vi "Delta_RH.vi"() -> ()   [LabVIEW 2019]
uses:
  <vilib>/Analysis/baseanly.llb/Mean (DBL).vi
  DeltaRamp_globals.vi
  Global 2.vi
  B_Globals.vi
  <vilib>/Analysis/NI_AALBase.lvlib
panel:
  in  "RW Delay":i32=50
  out "Exec Time [ms]":u32
  in  "Reading Delay [ms]":i32=100 min=5
  out "read buffer":string
  in  "B/T":bool
  in  "Smart Avs":bool=TRUE
  in  "Points":dbl=1.0
  out "PpP":dbl
  in  "Combo Box":string(combo)
  in  "Save":bool
  in  "Abort Delta":bool
  out "B [T]":dbl=0.49837
  in  "Arm":bool
  in  "Measure":bool
  in  "Comp":dbl=10.0
  in  "Delay":dbl=0.002
  in  "I_Max":dbl=0.00055
  out "T":cluster{"X":dbl[], "Y":dbl[]}[](graph)=[{"X"=[0.48596000000030654, 0.48632999999976745, 0.4888800000004717, 0.4914299999991856, 0.49799999999988437, 0.49837000000048626, 0.49799999999964834, 0.49764000000059827, 0.4972699999998548, 0.49799999999964706, 0.4976400000005962, 0.4979999999996451, 0.49764000000114167, 0.4987299999995217, 0.49837000000048276, 0.4979999999996453, 0.49764000000060443, 0.4980000000000499, 0.4983700000004744, 0.4979999999996602, 0.4983700000001006, 0.4979999999996734, 0.49764000000018094, 0.4979999999996305, 0.4976400000006558, 0.4979999999996311, 0.4976399999998779, 0.49799999999967304, 0.4983699999999628, 0.49799999999964784, 0.49764000000002906, 0.4983699999999084, 0.49799999999967276, 0.498370000000109, 0.4979999999996426, 0.4983700000001016, 0.4979999999996246, 0.4983700000001098, 0.4979999999996428, 0.4976400000006453], "Y"=[nan, nan, nan, nan, nan, nan, nan, nan, nan, nan, nan, nan, nan, nan, nan, nan, nan, nan, nan, nan, nan, nan, nan, nan, nan, nan, nan, nan, nan, nan, nan, nan, nan, nan, nan, nan, nan, nan, nan, nan]}] caption="XY Graph"
  in  "Reset":bool
  out "Spl T [K]":dbl=6.1992
  out "R [Ohm]":dbl=nan
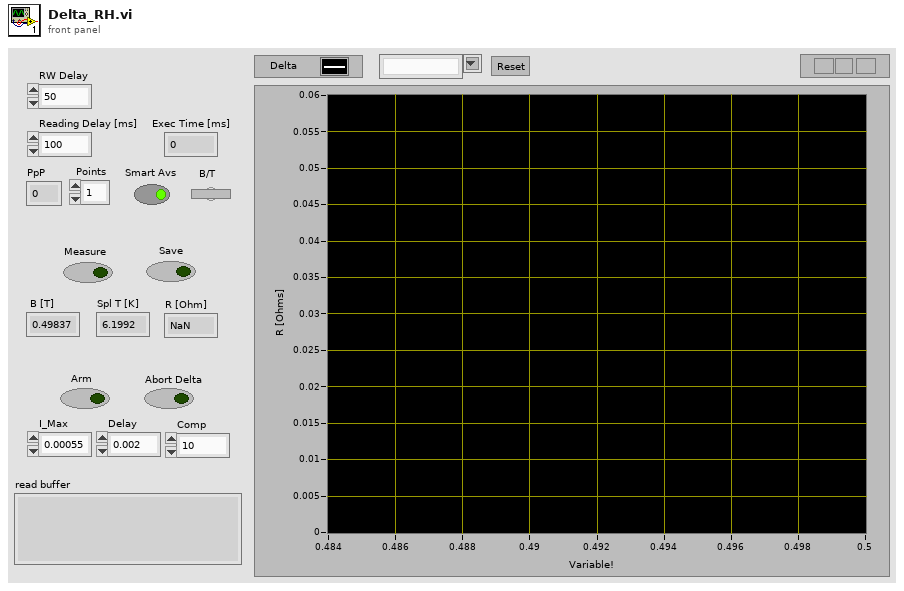
[diagram p1: front panel]
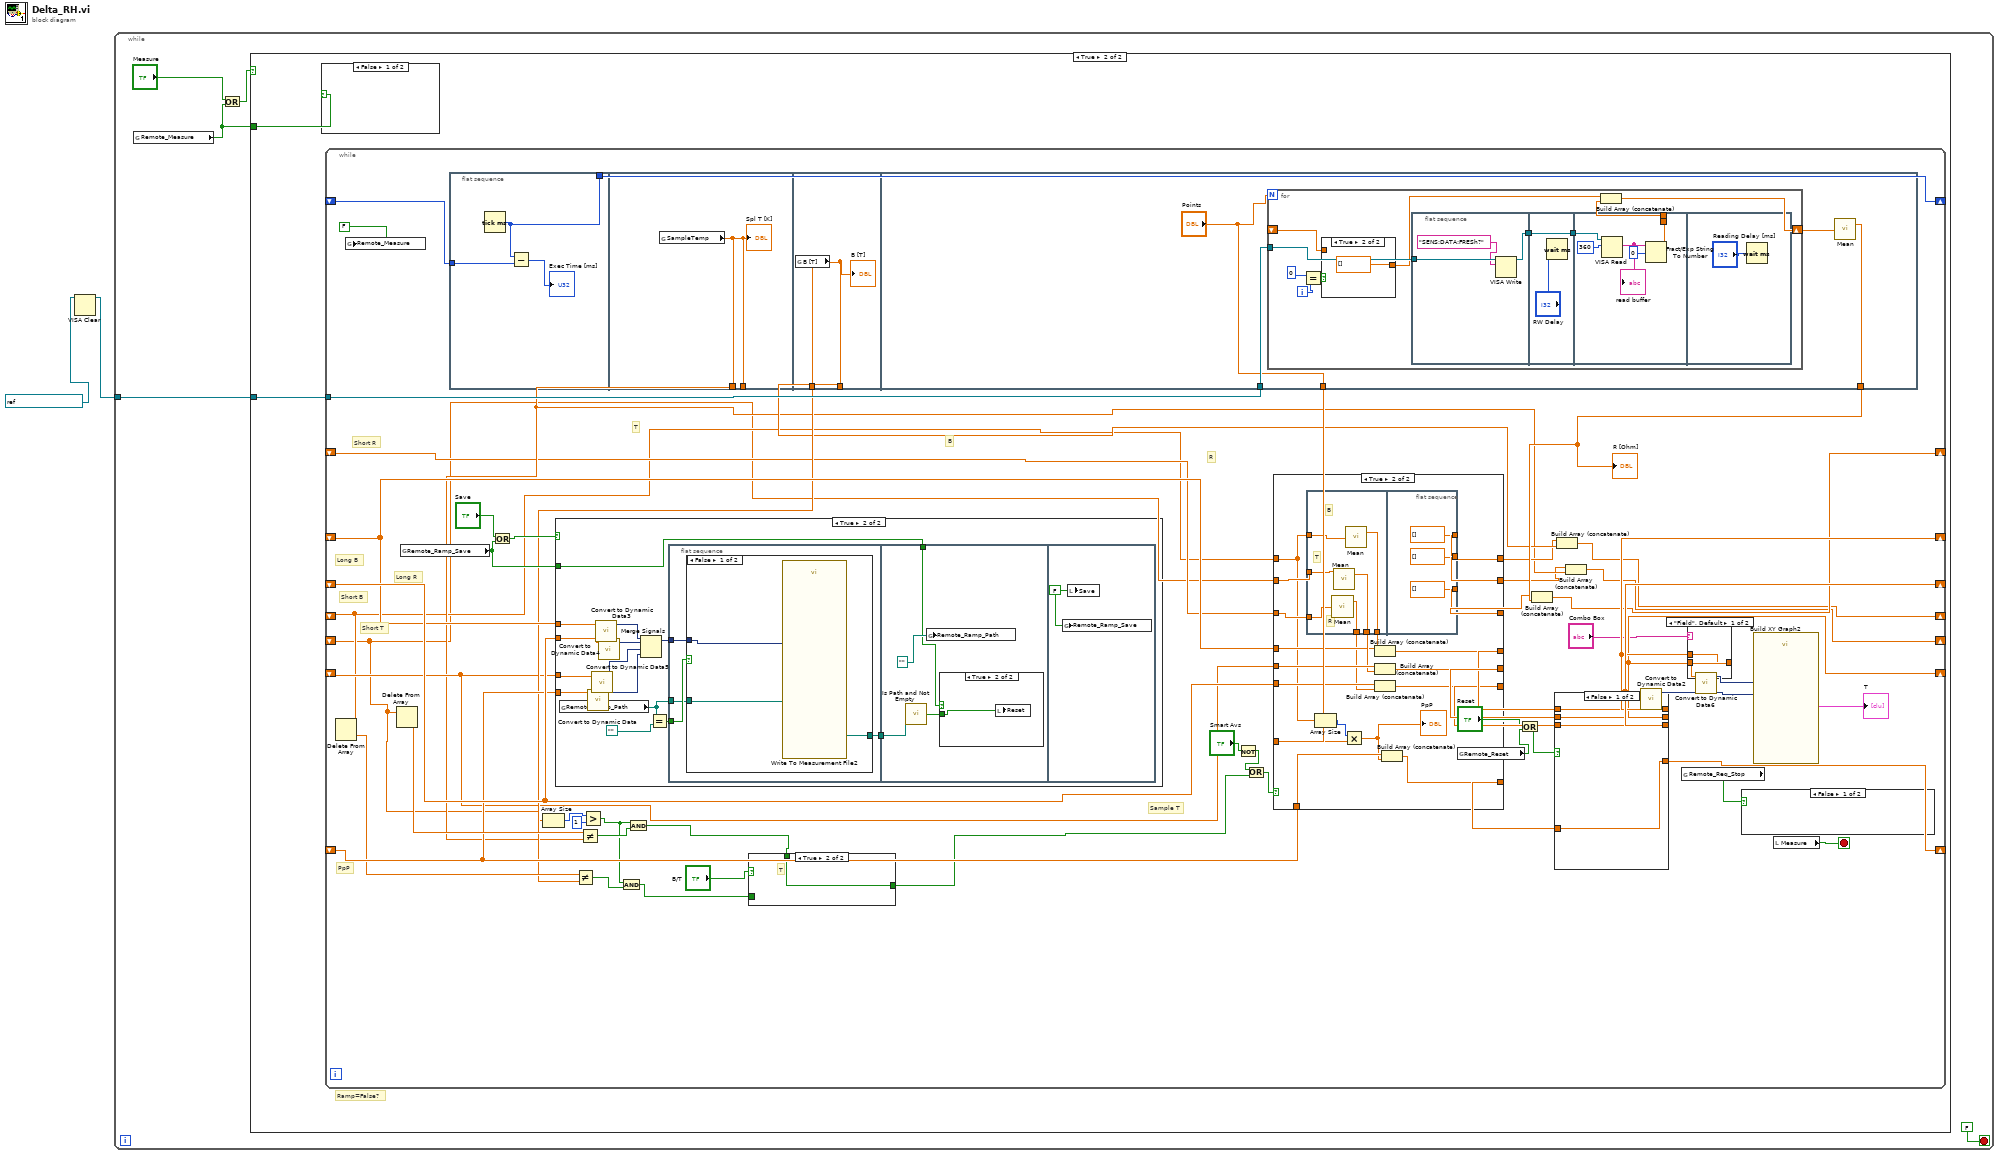
[diagram p0: block diagram]
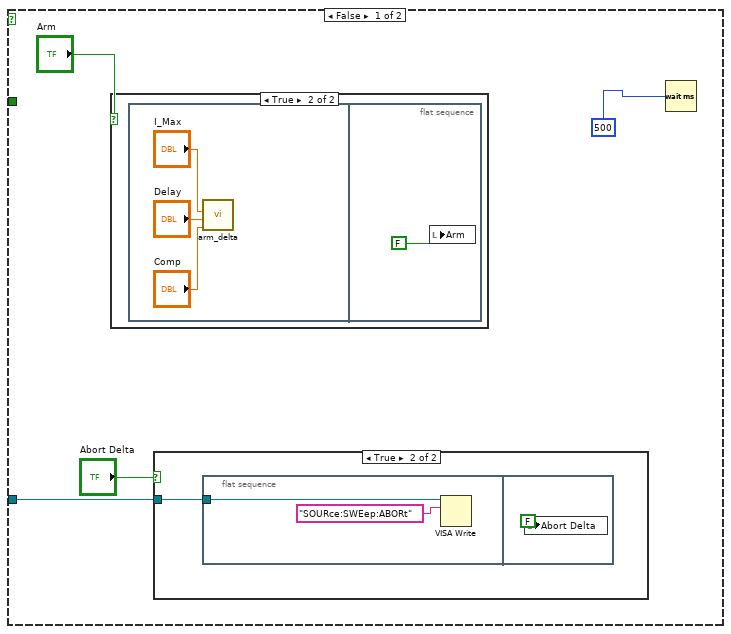
[diagram p2: hidden frame]
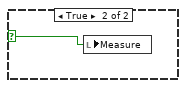
[diagram p5: hidden frame]
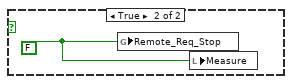
[diagram p7: hidden frame]
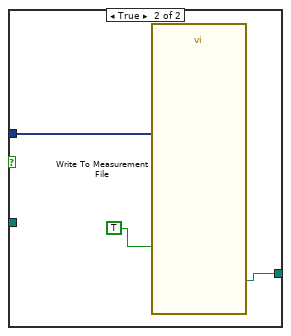
[diagram p11: hidden frame]
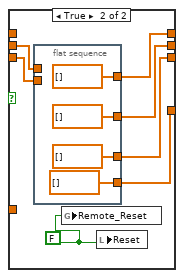
[diagram p14: hidden frame]
diagram:
  n1 = VISA Clear(VISA resource name=refnum<visa-resource-name> "GPIB1::20::INSTR" ("Keithley")) -> (VISA resource name out=w2:refnum<visa-resource-name>)  [unwired: 1 in, 1 out]
  n2 = while {
    tunnel: w2 -> [w6]
    stop <- FALSE stop-if-true
    n3 = global read "DeltaRamp_globals.vi" "Remote_Measure"() -> (w3:bool)
    n4 = Or(x="Measure", y=w3) -> (x .or. y?=w5:bool)
    n5 = case shown="True" w5 {
      tunnel: w6 -> [w9 w21]
      tunnel: w3 -> [_ w20]
      frame False {
        n6 = case shown="True" "Arm" {
          frame False {
          }
          frame True {
            n7 = flat-sequence {
              frame #0 {
                n8 = call "arm_delta.vi"("Compliance [V]"="Comp", "DELAY [sec]"="Delay", "I-HIGH [A]"="I_Max") -> ()  [unwired: 9 in]
              }
              frame #1 {
                n9 = local write "Arm"(FALSE) -> ()
              }
            }
          }
        }
        n10 = case shown="True" "Abort Delta" {
          tunnel: w9 -> [_ w12]
          frame False {
          }
          frame True {
            n11 = flat-sequence {
              tunnel: w12 -> [w14]
              frame #0 {
                n12 = VISA Write(VISA resource name=w14, write buffer="SOURce:SWEep:ABORt") -> ()  [unwired: 1 in, 3 out]
              }
              frame #1 {
                n13 = local write "Abort Delta"(FALSE) -> ()
              }
            }
          }
        }
        n14 = Wait (ms)(milliseconds to wait=500) -> ()  [unwired: 1 out]
      }
      frame True {
        # "Ramp=False?"
        n15 = case shown="False" w20 {
          selector: w20 -> [_ w22]
          frame False {
          }
          frame True {
            n16 = local write "Measure"(w22) -> ()
          }
        }
        n17 = while {
          shift-right: [w73] -> _
          shift-left: _ -> [w37]
          shift-right: [w78] -> _
          shift-left: _ -> [w66]
          tunnel: w21 -> [w56]
          shift-right: [w75] -> _
          shift-left: _ -> [w65]
          shift-right: [w28] -> _
          shift-left: _ -> [w25]
          shift-right: [w31] -> _
          shift-left: _ -> [w26]
          shift-right: [w34] -> _
          shift-left: _ -> [w27]
          shift-right: [w52] -> _
          shift-left: _ -> [w50]
          shift-right: [w23] -> _
          shift-left: _ -> [w24]
          stop <- w76 stop-if-true
          # "Short T"
          # "Short R"
          # "PpP"
          # "Short B"
          # "Long R"
          # "Long B"
          # "T"
          # "B"
          # "R"
          # "Sample T"
          n18 = Delete From Array(array=w26) -> (deleted portion=w44:dbl)  [unwired: 2 in, 1 out]
          n19 = global write "DeltaRamp_globals.vi" "Remote_Measure"(FALSE) -> ()
          n20 = Delete From Array(array=w25) -> (deleted portion=w70:dbl)  [unwired: 2 in, 1 out]
          n21 = global read "DeltaRamp_globals.vi" "Remote_Ramp_Save"() -> (w57:bool)
          n22 = flat-sequence {
            tunnel: w24 -> [w153]
            tunnel: [w151] -> w23
            tunnel: [w154] -> _
            tunnel: [w154] -> w30
            tunnel: [w155] -> w33
            tunnel: [w155] -> w38
            tunnel: w56 -> [w159]
            tunnel: [w157] -> w36
            tunnel: ["Points"] -> w46
            frame #0 {
              n23 = Tick Count (ms)() -> (millisecond timer value=w151:u32)
              n24 = Subtract(x=w151, y=w153) -> (x-y=→"Exec Time [ms]":u32)
            }
            frame #1 {
              n25 = global read "Global 2.vi" "SampleTemp"() -> (w154:dbl)
              "Spl T [K]" <- w154
            }
            frame #2 {
              n26 = global read "B_Globals.vi" "B [T]"() -> (w155:dbl)
              "B [T]" <- w155
            }
            frame #3 {
              n27 = for {
                N: "Points" -> [_]
                tunnel: w159 -> [w169]
                shift-right: [w168] -> w158
                shift-left: _ -> [w160]
                i -> [w162]
                n28 = Equal?(x=0, y=w162) -> (x = y?=w164:bool)
                n29 = case shown="True" w164 {
                  tunnel: [w170 dbl[] [] ("Numeric")] -> w161
                  tunnel: w160 -> [w170 _]
                  frame False {
                  }
                  frame True {
                  }
                }
                n30 = flat-sequence {
                  tunnel: w169 -> [w174]
                  tunnel: [w173] -> w165
                  tunnel: [w175] -> w166
                  tunnel: w165 -> [w175]
                  tunnel: [w179] -> _
                  tunnel: [w179] -> w167
                  tunnel: w166 -> [w178]
                  frame #0 {
                    n31 = VISA Write(VISA resource name=w174, write buffer="SENS:DATA:FRESh?" ("write buffer 2")) -> (VISA resource name out=w173:refnum<visa-resource-name>)  [unwired: 1 in, 2 out]
                  }
                  frame #1 {
                    n32 = Wait (ms)(milliseconds to wait="RW Delay") -> ()  [unwired: 1 out]
                  }
                  frame #2 {
                    n33 = VISA Read(VISA resource name=w178, byte count=u32 360) -> (read buffer=w177:string)  [unwired: 1 in, 3 out]
                    "read buffer" <- w177
                    n34 = Fract/Exp String To Number(string=w177, offset=0) -> (number=w179:dbl)  [unwired: 3 out]
                  }
                  frame #3 {
                    n35 = Wait (ms)(milliseconds to wait="Reading Delay [ms]") -> ()  [unwired: 1 out]
                  }
                }
                n36 = Build Array (concatenate)(w161, w167) -> (w168:dbl[])
              }
              n37 = call-poly <vilib>:"Mean.vi"("X"=w158) -> ("mean"=w157:dbl)  [unwired: 1 out]
            }
          }
          n38 = Or(x="Save", y=w57) -> (x .or. y?=w63:bool)
          n39 = Array Size(array=w25) -> (size(s)=w48:i32)
          n40 = case shown="True" w63 {
            tunnel: w65 -> [_ w133]
            tunnel: w66 -> [_ w131]
            tunnel: w37 -> [_ w129]
            tunnel: w57 -> [_ w123]
            tunnel: w50 -> [_ w122]
            frame False {
            }
            frame True {
              n41 = global read "DeltaRamp_globals.vi" "Remote_Ramp_Path"() -> (w125:path)
              n42 = call "Convert to Dynamic Data"("Array"=w122) -> ("Dynamic Data Type"=w121:dynamicdata)  [unwired: 3 in]
              n43 = call "Convert to Dynamic Data5"("Array"=w129) -> ("Dynamic Data Type"=w128:dynamicdata)  [unwired: 3 in]
              n44 = call "Convert to Dynamic Data3"("Array"=w133) -> ("Dynamic Data Type"=w132:dynamicdata)  [unwired: 3 in]
              n45 = call "Convert to Dynamic Data4"("Array"=w131) -> ("Dynamic Data Type"=w130:dynamicdata)  [unwired: 3 in]
              n46 = Merge Signals(w132, w130, w128, w121) -> (w134:dynamicdata)
              n47 = Equal?(x=w125, y=path "") -> (x = y?=w126:bool)
              n48 = flat-sequence {
                tunnel: w134 -> [w138]
                tunnel: w126 -> [w137]
                tunnel: w125 -> [w136]
                tunnel: [w135] -> w124
                tunnel: w124 -> [w147]
                tunnel: w123 -> [w146]
                frame #0 {
                  n49 = case shown="False" w137 {
                    tunnel: w138 -> [w141 w143]
                    tunnel: w136 -> [w140 _]
                    tunnel: [w139 w142] -> w135
                    frame False {
                      n50 = call "Write To Measurement File2"("Signals"=w141, "Filename"=w140) -> ("Filename Out"=w139:path)  [unwired: 15 in, 2 out]
                    }
                    frame True {
                      n51 = call "Write To Measurement File"("Signals"=w143, "Reset"=TRUE) -> ("Filename Out"=w142:path)  [unwired: 15 in, 2 out]
                    }
                  }
                }
                frame #1 {
                  n52 = call <vilib>:"Is Path and Not Empty.vi"("path"=w147) -> ("Is Path and Not Empty?"=w145:bool)  [unwired: 4 in]
                  n53 = global write "DeltaRamp_globals.vi" "Remote_Ramp_Path"(path "") -> ()
                  n54 = case shown="True" w146 {
                    tunnel: w145 -> [_ w149]
                    frame False {
                    }
                    frame True {
                      n55 = local write "Reset"(w149) -> ()
                    }
                  }
                }
                frame #2 {
                  w150 = FALSE
                  n56 = global write "DeltaRamp_globals.vi" "Remote_Ramp_Save"(w150) -> ()
                  n57 = local write "Save"(w150) -> ()
                }
              }
            }
          }
          n58 = Not Equal?(x=w44, y=w38) -> (x != y?=w42:bool)
          n59 = Not Equal?(x=w70, y=w30) -> (x != y?=w47:bool)
          n60 = Greater?(x=w48, y=1) -> (0:w43:bool)
          n61 = And(x=w43, y=w42) -> (x .and. y?=w41:bool)
          n62 = And(x=w43, y=w47) -> (x .and. y?=w40:bool)
          n63 = case shown="True" "B/T" {
            tunnel: w41 -> [w80 _]
            tunnel: w40 -> [_ w81]
            tunnel: [w80 w81] -> w39
            frame False {
              # "B"
            }
            frame True {
              # "T"
            }
          }
          n64 = Not(x="Smart Avs") -> (.not. x?=w54:bool)
          n65 = Or(x=w54, y=w39) -> (x .or. y?=w53:bool)
          n66 = case shown="True" w53 {
            tunnel: w27 -> [w87 w106]
            tunnel: w26 -> [w88 w95]
            tunnel: w25 -> [w89 w105]
            tunnel: [w89 w109] -> w29
            tunnel: [w88 w108] -> w32
            tunnel: [w87 w107] -> w35
            tunnel: w37 -> [w85 w104]
            tunnel: [w85 w102] -> w69
            tunnel: w65 -> [w84 w101]
            tunnel: [w84 w100] -> w68
            tunnel: w66 -> [w86 w99]
            tunnel: [w86 w97] -> w67
            tunnel: [w83 w94] -> w51
            tunnel: w50 -> [w83 w93]
            tunnel: w46 -> [_ w90]
            frame False {
              # "R"
              # "T"
              # "B"
            }
            frame True {
              n67 = flat-sequence {
                tunnel: w106 -> [w115]
                tunnel: w105 -> [w112]
                tunnel: w95 -> [w111]
                tunnel: [w113] -> w103
                tunnel: [w110] -> w96
                tunnel: [w114] -> w98
                tunnel: [dbl[] []] -> w107
                tunnel: [dbl[] []] -> w109
                tunnel: [dbl[] []] -> w108
                frame #0 {
                  # "T"
                  # "R"
                  # "B"
                  n68 = call-poly <vilib>:"Mean.vi"("X"=w115) -> ("mean"=w114:dbl)  [unwired: 1 out]
                  n69 = call-poly <vilib>:"Mean.vi"("X"=w112) -> ("mean"=w113:dbl)  [unwired: 1 out]
                  n70 = call-poly <vilib>:"Mean.vi"("X"=w111) -> ("mean"=w110:dbl)  [unwired: 1 out]
                }
                frame #1 {
                }
              }
              n71 = Array Size(array=w95) -> (size(s)=w92:i32)
              n72 = Multiply(x=w92, y=w90) -> (x*y=w91:dbl)
              "PpP" <- w91
              n73 = Build Array (concatenate)(w101, w96) -> (w100:dbl[])
              n74 = Build Array (concatenate)(w104, w103) -> (w102:dbl[])
              n75 = Build Array (concatenate)(w99, w98) -> (w97:dbl[])
              n76 = Build Array (concatenate)(w93, w91) -> (w94:dbl[])
            }
          }
          n77 = global read "DeltaRamp_globals.vi" "Remote_Reset"() -> (w61:bool)
          n78 = Or(x="Reset", y=w61) -> (x .or. y?=w59:bool)
          n79 = Build Array (concatenate)(w35, w36) -> (w34:dbl[])
          n80 = case shown="False" w59 {
            tunnel: w69 -> [w186 w193]
            tunnel: [w186 w192] -> w73
            tunnel: w67 -> [w185 w191]
            tunnel: [w185 w190] -> w78
            tunnel: [w184 w189] -> w75
            tunnel: w68 -> [w184 _]
            tunnel: [w183 w187] -> w52
            tunnel: w51 -> [w183 _]
            frame False {
            }
            frame True {
              w188 = FALSE
              n81 = flat-sequence {
                tunnel: w193 -> [_]
                tunnel: w191 -> [_]
                tunnel: [dbl[] []] -> w190
                tunnel: [dbl[] []] -> w192
                tunnel: [dbl[] []] -> w189
                tunnel: [dbl[] [] ("Numeric")] -> w187
                frame #0 {
                }
              }
              n82 = global write "DeltaRamp_globals.vi" "Remote_Reset"(w188) -> ()
              n83 = local write "Reset"(w188) -> ()
            }
          }
          n84 = Build Array (concatenate)(w32, w33) -> (w31:dbl[])
          n85 = Build Array (concatenate)(w29, w30) -> (w28:dbl[])
          n86 = call "Convert to Dynamic Data2"("Array"=w78) -> ("Dynamic Data Type"=w79:dynamicdata)  [unwired: 3 in]
          n87 = global read "DeltaRamp_globals.vi" "Remote_Req_Stop"() -> (w58:bool)
          n88 = case shown="\"Field\", Default" "Combo Box" {
            tunnel: w75 -> [w119 _]
            tunnel: [w119 w120] -> w74
            tunnel: w73 -> [_ w120]
            frame "Field", Default {
            }
            frame "Temp" {
            }
          }
          n89 = call "Convert to Dynamic Data6"("Array"=w74) -> ("Dynamic Data Type"=w72:dynamicdata)  [unwired: 3 in]
          n90 = case shown="False" w58 {
            frame False {
            }
            frame True {
              w82 = FALSE
              n91 = global write "DeltaRamp_globals.vi" "Remote_Req_Stop"(w82) -> ()
              n92 = local write "Measure"(w82) -> ()
            }
          }
          n93 = call "Build XY Graph2"("Y Input"=w79, "X Input"=w72) -> ("XY Graph"=→"T":cluster{"X":dbl[], "Y":dbl[]}[])  [unwired: 8 in, 1 out]
          n94 = local read "Measure"() -> (w76:bool)
          "R [Ohm]" <- w36
        }
      }
    }
  }
